vi "Clear Query.vi"(11 "URI in":refnum<class "URI.lvclass">) -> (3 "URI out":refnum<class "URI.lvclass">)   [LabVIEW 2020, in "URI.lvlib" / "URI.lvclass"]
uses:
  URI.lvclass
  URI.lvclass/URI.ctl
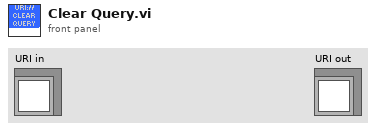
[diagram p1: front panel]
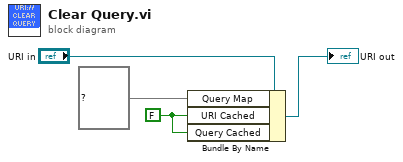
[diagram p0: block diagram]
diagram:
  w1 = FALSE ("String Cached")
  n1 = Bundle By Name(cluster="URI in", "Query Map"=map{string, string} {}, "URI Cached"=w1, "Query Cached"=w1) -> (→"URI out":refnum<class "URI.lvclass">)
